vi "Disconnect.vi"(8 "error in (no error)":errorcluster, 11 "reference in":refnum<class "Camera_Sim.lvclass">) -> (0 "error out":errorcluster, 3 "reference out":refnum<class "Camera_Sim.lvclass">)   [LabVIEW 2017, in "Camera_Sim.lvclass"]
doc: "Closes connection to an IMAQ camera"
uses:
  Camera_Sim.lvclass
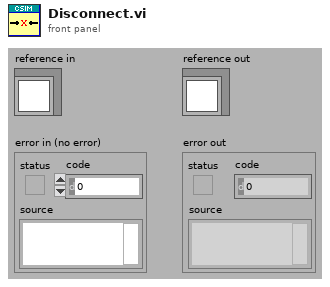
[diagram p1: front panel]
types:
  T1 = typedef "CameraSim.lvclass/ObjectAttributes.ctl" = cluster{"Connected":bool, "Image Out":T2, "Frame Number":u32, "Path":path}
  T2 = typedef "IMAQ Image.ctl" = refnum<image>
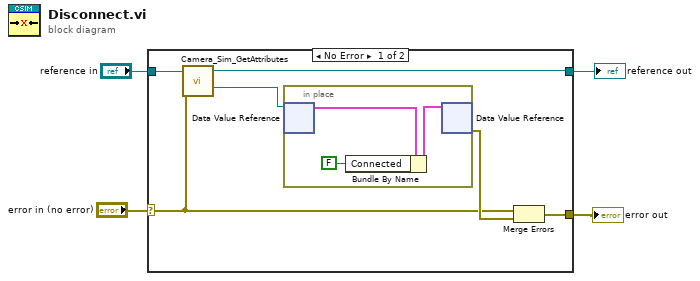
[diagram p0: block diagram]
diagram:
  n1 = case shown="No Error" "error in (no error)" {
    selector: "error in (no error)" -> [w6 w15]
    tunnel: [w5 w15] -> w3
    tunnel: [w8 w14] -> w1
    tunnel: "reference in" -> [w10 w14]
    frame No Error {
      n2 = call "Camera_Sim_GetAttributes.vi"("reference in"=w10, "error in (no error)"=w6) -> ("reference out"=w8:refnum<class "Camera_Sim.lvclass">, "DataRef"=w7:refnum<data-value>)  [unwired: 10 in, 2 out]
      n3 = in-place {
        n4 = in-place-dvr #1(w7) -> (w13:T1)  [unwired: 1 out]
        n5 = Bundle By Name(cluster=w13, "Connected"=FALSE) -> (w12:T1)
        n6 = in-place-dvr #1(w12) -> (w9:errorcluster)  [unwired: 1 out]
      }
      n7 = Merge Errors(w6, w9) -> (w5:errorcluster)
    }
    frame Error {
    }
  }
  "error out" <- w3
  "reference out" <- w1
